vi "外部窗口显示.vi"   [LabVIEW 2018]
uses:
  <vilib>/vision/NI_Vision_Development_Module.lvlib
types:
  T1 = enum32{"Gray", "Binary", "Gradient", "Rainbow", "Temperature"}
  T2 = typedef "Image Type" = u32
  T3 = typedef "IMAQ Image.ctl" = refnum<image>
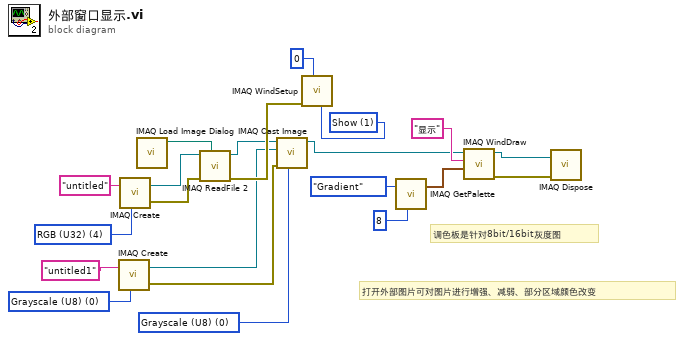
[diagram p0: block diagram]
diagram:
  w6 = T2 0 items=["Grayscale (U8)", "Grayscale (I16)", "Grayscale (SGL)", "Complex (CSG)", "RGB (U32)", "HSL (U32)", "RGB (U64)", "Grayscale (U16)"] ("Image Type")
  w7 = T2 4 items=["Grayscale (U8)", "Grayscale (I16)", "Grayscale (SGL)", "Complex (CSG)", "RGB (U32)", "HSL (U32)", "RGB (U64)", "Grayscale (U16)"] ("Image Type")
  w8 = T2 0 items=["Grayscale (U8)", "Grayscale (I16)", "Grayscale (SGL)", "Complex (CSG)", "RGB (U32)", "HSL (U32)", "RGB (U64)", "Grayscale (U16)"] ("Image Type")
  w4 = 1 items=["Hide", "Show", "No change"] ("Scrollbars (No change)")
  # "打开外部图片可对图片进行增强、减弱、部分区域颜色改变"
  # "调色板是针对8bit/16bit灰度图"
  n1 = call "IMAQ Create"("Image Name"="untitled1", "Image Type"=w6) -> ("New Image"=w10:T3, "error out"=w9:errorcluster)  [unwired: 3 in]
  n2 = call "IMAQ Create"("Image Name"="untitled", "Image Type"=w7) -> ("New Image"=w19:T3, "error out"=w18:errorcluster)  [unwired: 3 in]
  n3 = call "IMAQ Load Image Dialog"() -> ("Path"=w21:path)  [unwired: 9 in, 2 out]
  n4 = call "IMAQ ReadFile 2"("File Path"=w21, "error in (no error)"=w18, "Image"=w19) -> ("error out"=w16:errorcluster, "Image Out"=w12:T3)  [unwired: 4 in, 3 out]
  n5 = call "IMAQ Cast Image"("Image Type"=w8, "error in (no error)"=w9, "Image Dst"=w10, "Image Src"=w12) -> ("Image Dst Out"=w5:T3)  [unwired: 6 in, 1 out]
  n6 = call "IMAQ WindSetup"("Scrollbars (No change)"=w4, "Window Number (0...15)"=0, "error in (no error)"=w16) -> ()  [unwired: 8 in, 1 out]
  n7 = call "IMAQ GetPalette"("Palette Number (gray)"=T1."Gradient", "Bit Depth"=u32 8) -> ("Color Palette"=w3:cluster{"Red":u8, "Green":u8, "Blue":u8}[])  [unwired: 3 in, 1 out]
  n8 = call "IMAQ WindDraw"("Color Palette"=w3, "Title"="显示", "Image"=w5) -> ("error out"=w13:errorcluster, "Image Out (duplicate)"=w14:T3)  [unwired: 7 in]
  n9 = call "IMAQ Dispose"("Image"=w14, "error in (no error)"=w13) -> ()  [unwired: 4 in, 1 out]
